vi "XNET Reflective Memory Timing Source VI.vi"(8 "error in (no error)":errorcluster, 10 "Loop Time (usec)":u32, 11 "Device Ref":T1=18446744073709551615 format="%.0x") -> (0 "error out":errorcluster, 1 "Primary Control Loop dt":i64, 2 "Actual Loop Rate (Hz)":dbl, 3 "Timing Source Name":string)   [LabVIEW 2010, in "XNET Reflective Memory Custom Device.lvlib"]
uses:
  XNET Reflective Memory Custom Device.lvlib
  <vilib>/NI VeriStand/Custom Device API/Custom Device Item Ref.ctl
  RT DATA.ctl
  Single Category.ctl
  BeforeAfter.ctl
  <vilib>/NI VeriStand/Custom Device API/Data Reference.ctl
  Global.vi
  <vilib>/NI VeriStand/Custom Device API/Get Item Property (Boolean).vi
  <vilib>/xnet/xnet.llb/XNET Create Timing Source (FlexRay Cycle).vi
  <vilib>/NI Veristand/Custom Device API/Custom Device API.lvlib
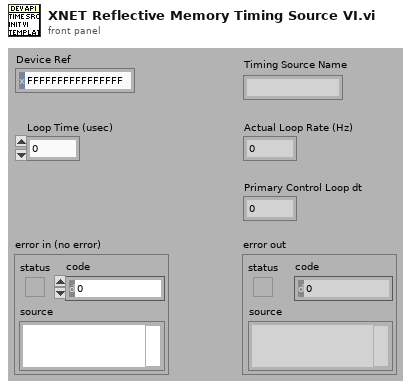
[diagram p1: front panel]
types:
  T1 = typedef "Custom Device API.lvlib/Custom Device Item Ref.ctl" = u64
  T2 = typedef "XNET Reflective Memory Custom Device.lvlib/RT DATA.ctl" = cluster{" Inputs":T3, "Outputs":T3, "Internal Iteration":i32, "Device Error":errorcluster}
  T3 = typedef "XNET Reflective Memory Custom Device.lvlib/Single Category.ctl" = cluster{"Vals":dbl[], "When":T4[], "Data Refs":T5[], "Session":refnum<k21>}
  T4 = typedef "XNET Reflective Memory Custom Device.lvlib/BeforeAfter.ctl" = enum16{"Before", "After"}
  T5 = typedef "Custom Device API.lvlib/Data Reference.ctl" = i32
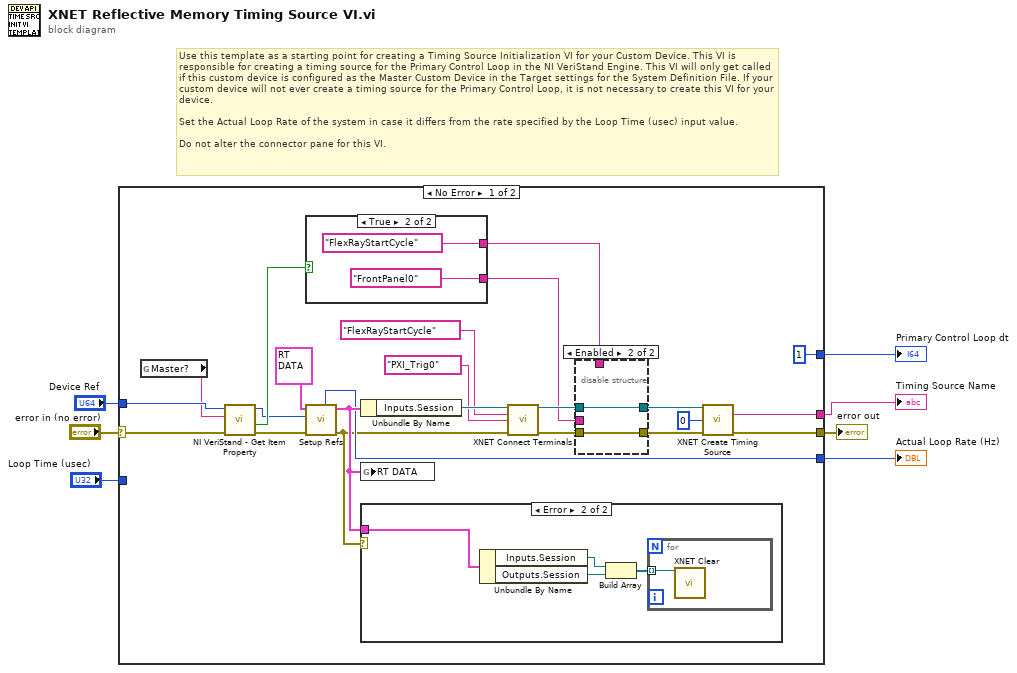
[diagram p0: block diagram]
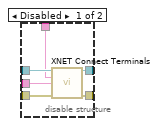
[diagram p2: hidden frame]
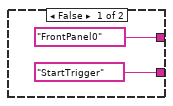
[diagram p3: hidden frame]
diagram:
  # "Use this template as a starting point for creating a Timing Source Initialization VI for your Custom Device. This VI is responsible for creating a timing source for the Primary Control Loop in the NI VeriStand Engine. This VI will only get called if this custom device is configured as the Master Custom Device in the Target settings for the System Definition File. If your custom device will not ever create a timing source for the Primary Control Loop, it is not necessary to create this VI for your device.\n\nSet the Actual Loop Rate of the system in case it differs from the rate specified by the Loop Time (usec) input value.\n\nDo not alter the connector pane for this VI."
  n1 = case shown="No Error" "error in (no error)" {
    selector: "error in (no error)" -> [w19 w48]
    tunnel: [w25 w48] -> w6
    tunnel: "Loop Time (usec)" -> [_ _]
    tunnel: [w26 _] -> w3
    tunnel: [w24 _] -> w2
    tunnel: [i64 1 ("Primary Control Loop dt") _] -> w1
    tunnel: "Device Ref" -> [w18 _]
    frame No Error {
      n2 = global read "Global.vi" "Master?"() -> (w16:string)
      n3 = call-poly <vilib>:"NI VeriStand - Get Item Property.vi"("error in (no error)"=w19, "Property Name"=w16, "Item Ref in"=w18) -> ("error out"=w17:errorcluster, "Value"=w15:bool, "Item Ref out"=w14:T1)  [unwired: 5 in, 1 out]
      n4 = case shown="True" w15 {
        tunnel: [tag "StartTrigger" ("source terminal") tag "FrontPanel0" ("source terminal")] -> w9
        tunnel: [tag "FrontPanel0" ("source terminal") tag "FlexRayStartCycle" ("source terminal")] -> w8
        frame False {
        }
        frame True {
        }
      }
      n5 = call "Setup Refs.vi"("error in (no error)"=w17, "Device Reference in"=w14, "RT Data In"=T2 {" Inputs"={"Vals"=[], "When"=[], "Data Refs"=[], "Session"=""}, "Outputs"={"Vals"=[], "When"=[], "Data Refs"=[], "Session"=""}, "Internal Iteration"=0, "Device Error"={"status"=FALSE, "code"=0, "source"=""}}) -> ("error out"=w23:errorcluster, "RT Data Out"=w27:T2, "Hz"=w26:u32)  [unwired: 6 in]
      n6 = Unbundle By Name(w27) -> ("Inputs.Session"=w22:refnum<k21>)
      n7 = global write "Global.vi" "RT DATA"(w27) -> ()
      n8 = case shown="Error" w23 {
        tunnel: w27 -> [_ w46]
        frame No Error {
        }
        frame Error {
          n9 = Unbundle By Name(w46) -> ("Inputs.Session"=w44:refnum<k21>, "Outputs.Session"=w45:refnum<k21>)
          n10 = Build Array(w44, w45) -> (w43:refnum<k21>[])
          n11 = for {
            tunnel: w43 -> [w47] mode=indexing
            n12 = call <vilib>:"XNET Clear.vi"("session in"=w47) -> ()  [unwired: 14 in, 1 out]
          }
        }
      }
      n13 = call <vilib>:"XNET Connect Terminals.vi"("session in"=w22, "source terminal"=tag "FlexRayStartCycle", "destination terminal"=tag "PXI_Trig0" ("source terminal"), "error in (no error)"=w23) -> ("session out"=w10:refnum<k21>, "error out"=w11:errorcluster)  [unwired: 10 in]
      n14 = disable-structure shown="Enabled" {
        disable-tunnel: [w36 w38] -> w13
        disable-tunnel: [w35 w37] -> w12
        disable-tunnel: w11 -> [w34 w37]
        disable-tunnel: w10 -> [w33 w38]
        disable-tunnel: w9 -> [w32 _]
        disable-tunnel: w8 -> [w31 _]
        frame Disabled {
          n15 = call <vilib>:"XNET Connect Terminals.vi"("session in"=w33, "source terminal"=w31, "destination terminal"=w32, "error in (no error)"=w34) -> ("session out"=w36:refnum<k21>, "error out"=w35:errorcluster)  [unwired: 10 in]
        }
        frame Enabled {
        }
      }
      n16 = call-poly <vilib>:"XNET Create Timing Source.vi"("session in"=w13, "macrotick offset"=u32 0, "error in (no error)"=w12) -> ("timing source out"=w24:string, "error out"=w25:errorcluster)  [unwired: 10 in, 1 out]
    }
    frame Error {
    }
  }
  "error out" <- w6
  "Timing Source Name" <- w2
  "Actual Loop Rate (Hz)" <- w3
  "Primary Control Loop dt" <- w1
